vi "士兵升变.vi"(2 "选项":enum16{"士兵", "骑士", "主教", "战车", "皇后"}(ring), 3 "到达的Y":u8, 4 "到达的X":u8, 5 "输入的棋盘":T1) -> (0 "输出棋盘":T1, 1 "数值":u8)   [LabVIEW 2017]
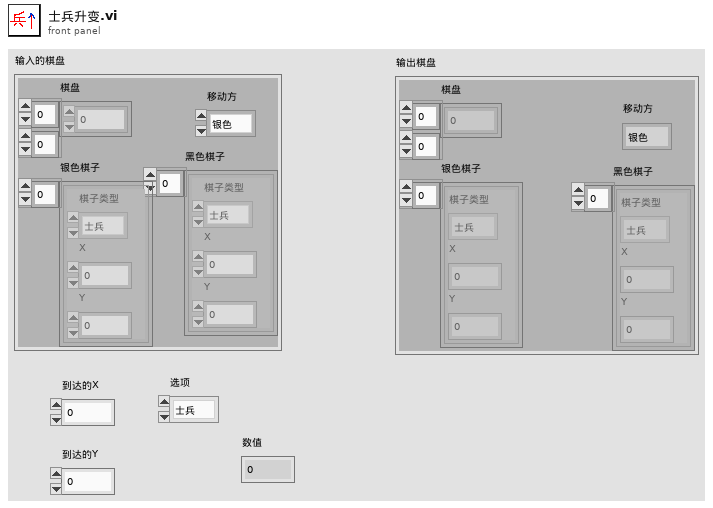
[diagram p1: front panel]
types:
  T1 = cluster{"棋盘":u16[][], "银色棋子":cluster{"棋子类型":enum16{"士兵", "骑士", "主教", "战车", "皇后", "国王", "空"}, "X":u8, "Y":u8}[], "黑色棋子":cluster{"棋子类型":enum16{"士兵", "骑士", "主教", "战车", "皇后", "国王", "空"}, "X":u8, "Y":u8}[], "移动方":enum16{"银色", "黑色"}}
  T2 = cluster{"棋子类型":enum16{"士兵", "骑士", "主教", "战车", "皇后", "国王", "空"}, "X":u8, "Y":u8}[]
  T3 = cluster{"y":enum16{"士兵", "骑士", "主教", "战车", "皇后", "国王", "空"}, "到达的X":u8, "到达的Y":u8}
  T4 = cluster{"棋子类型":enum16{"士兵", "骑士", "主教", "战车", "皇后", "国王", "空"}, "到达的X":u8, "到达的Y":u8}
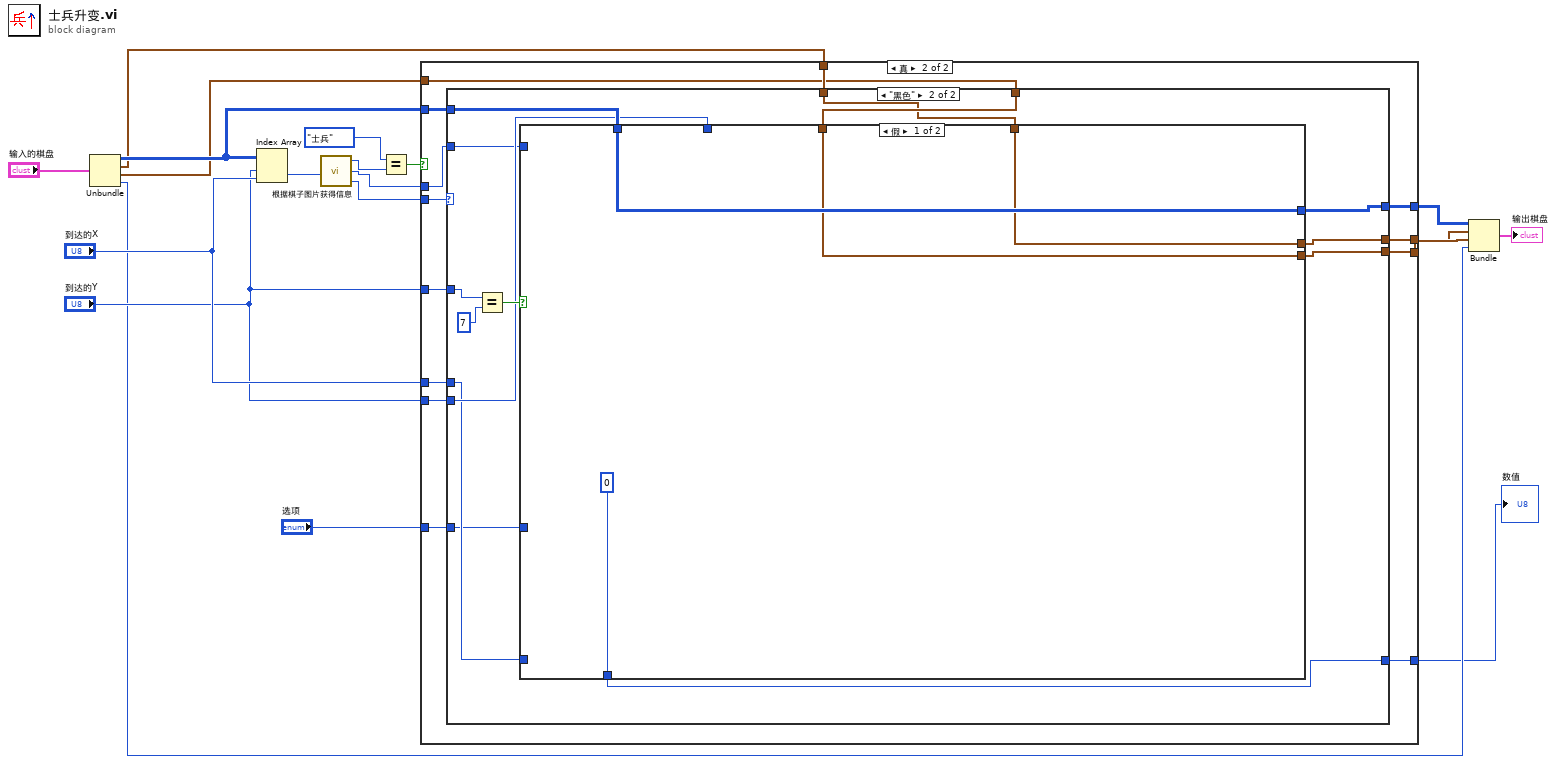
[diagram p0: block diagram]
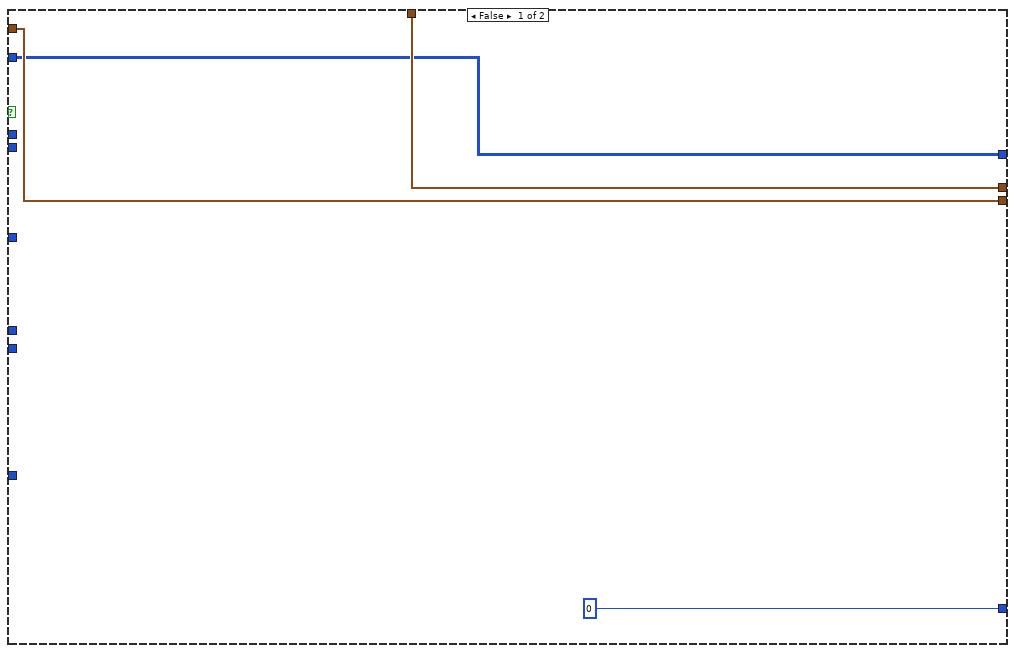
[diagram p2: hidden frame]
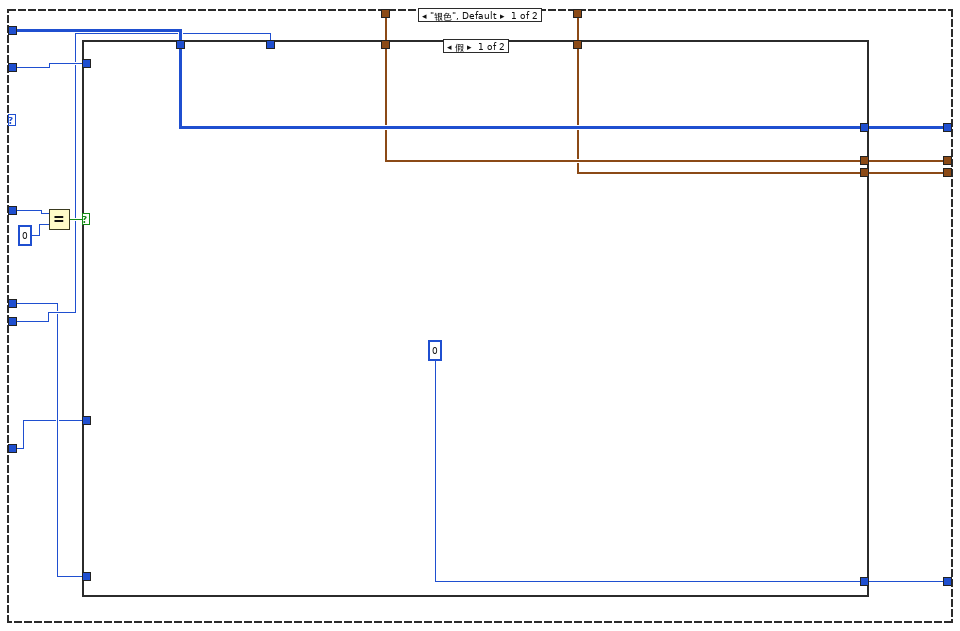
[diagram p3: hidden frame]
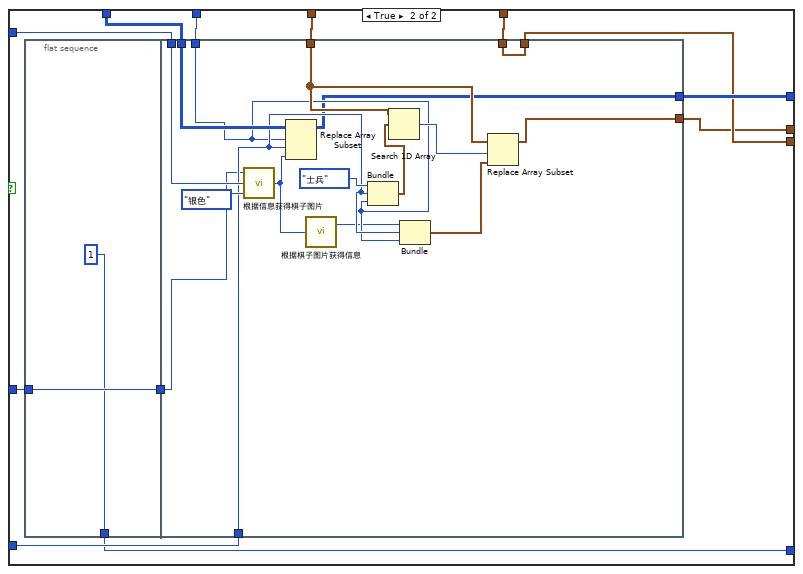
[diagram p4: hidden frame]
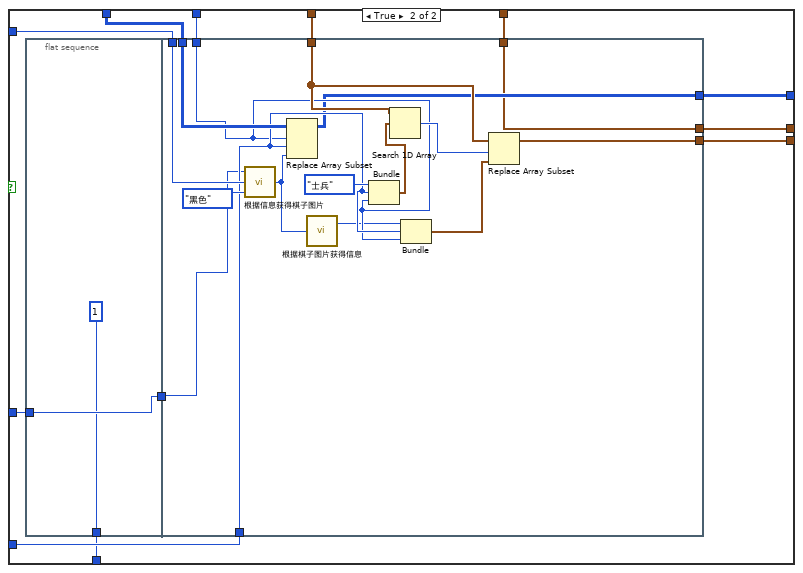
[diagram p5: hidden frame]
diagram:
  n1 = Unbundle("输入的棋盘") -> ("棋盘"=w14:u16[][], "银色棋子"=w9:T2, "黑色棋子"=w8:T2, "移动方"=w6:enum16{"银色", "黑色"})
  n2 = Index Array(array=w14, index (row)="到达的Y", index (col)="到达的X") -> (element=w18:u16)
  n3 = call "根据棋子图片获得信息.vi"("棋子"=w18) -> ("棋子类型"=w17:enum16{"士兵", "骑士", "主教", "战车", "皇后", "国王", "空"}, "背景颜色"=w11:enum16{"白色", "绿色"}, "棋子颜色"=w10:enum16{"银色", "黑色"})
  n4 = Equal?(x=enum16{"士兵", "骑士", "主教", "战车", "皇后", "国王", "空"}."士兵" ("y"), y=w17) -> (x = y?=w15:bool)
  n5 = case shown="真" w15 {
    tunnel: w10 -> [_ w36]
    tunnel: "到达的Y" -> [_ w35]
    tunnel: w14 -> [w21 w34]
    tunnel: "到达的X" -> [_ w33]
    tunnel: "到达的Y" -> [_ w32]
    tunnel: w11 -> [_ w31]
    tunnel: w9 -> [w23 w30]
    tunnel: w8 -> [w22 w29]
    tunnel: [w22 w27] -> w4
    tunnel: [w21 w28] -> w7
    tunnel: [w23 w26] -> w3
    tunnel: "选项" -> [_ w25]
    tunnel: [0 w24] -> w1
    frame False {
    }
    frame True {
      n6 = case shown="\"黑色\"" w36 {
        tunnel: w35 -> [w50 w97]
        tunnel: w34 -> [w47 w95]
        tunnel: w33 -> [w44 w92]
        tunnel: w32 -> [w45 w94]
        tunnel: w31 -> [w46 w93]
        tunnel: w30 -> [w43 w90]
        tunnel: w29 -> [w42 w91]
        tunnel: [w40 w87] -> w27
        tunnel: [w41 w89] -> w28
        tunnel: [w39 w88] -> w26
        tunnel: w25 -> [w38 w86]
        tunnel: [w37 w85] -> w24
        frame "银色", Default {
          n7 = Equal?(x=w50, y=u8 0) -> (x = y?=w48:bool)
          n8 = case shown="假" w48 {
            tunnel: w47 -> [w54 w66]
            tunnel: w46 -> [_ w65]
            tunnel: w45 -> [_ w64]
            tunnel: w44 -> [_ w63]
            tunnel: w43 -> [w53 w62]
            tunnel: w42 -> [w52 w61]
            tunnel: [w52 w59] -> w40
            tunnel: [w54 w60] -> w41
            tunnel: [w53 w58] -> w39
            tunnel: w38 -> [_ w56]
            tunnel: [0 w55] -> w37
            frame False {
            }
            frame True {
              n9 = flat-sequence {
                tunnel: [w68] -> w57
                tunnel: w56 -> [w68]
                tunnel: [1] -> w55
                tunnel: w66 -> [w84]
                tunnel: w65 -> [w83]
                tunnel: w64 -> [w75]
                tunnel: w63 -> [w76]
                tunnel: w62 -> [w79]
                tunnel: w61 -> [w71]
                tunnel: [w71] -> w59
                tunnel: [w72] -> w60
                tunnel: [w70] -> w58
                tunnel: w57 -> [w69]
                frame #0 {
                }
                frame #1 {
                  n10 = call "根据信息获得棋子图片.vi"("棋子颜色"=enum16{"银色", "黑色"}."银色", "背景颜色"=w83, "棋子类型"=w69) -> ("棋子"=w77:u16)
                  n11 = Replace Array Subset(array=w84, new element=w77, index (row)=w75, index (col)=w76) -> (w72:u16[][])
                  n12 = call "根据棋子图片获得信息.vi"("棋子"=w77) -> ("棋子类型"=w74:enum16{"士兵", "骑士", "主教", "战车", "皇后", "国王", "空"})  [unwired: 2 out]
                  n13 = Bundle("y"=enum16{"士兵", "骑士", "主教", "战车", "皇后", "国王", "空"}."士兵", "到达的X"=w76, "到达的Y"=w75) -> (w80:T3)  [unwired: 1 in]
                  n14 = Search 1D Array(1D array=w79, element=w80) -> (index of element=w78:i32)  [unwired: 1 in]
                  n15 = Bundle("棋子类型"=w74, "到达的X"=w76, "到达的Y"=w75) -> (w73:T4)  [unwired: 1 in]
                  n16 = Replace Array Subset(array=w79, new element=w73, index=w78) -> (w70:T2)
                }
              }
            }
          }
        }
        frame "黑色" {
          n17 = Equal?(x=w97, y=u8 7) -> (x = y?=w98:bool)
          n18 = case shown="假" w98 {
            tunnel: w95 -> [w102 w114]
            tunnel: w93 -> [_ w113]
            tunnel: w94 -> [_ w112]
            tunnel: w92 -> [_ w111]
            tunnel: w91 -> [w100 w110]
            tunnel: w90 -> [w101 w109]
            tunnel: [w100 w108] -> w87
            tunnel: [w102 w107] -> w89
            tunnel: [w101 w106] -> w88
            tunnel: w86 -> [_ w105]
            tunnel: [0 w103] -> w85
            frame False {
            }
            frame True {
              n19 = flat-sequence {
                tunnel: w105 -> [w116]
                tunnel: [w116] -> w104
                tunnel: [1] -> w103
                tunnel: w114 -> [w132]
                tunnel: w113 -> [w131]
                tunnel: w112 -> [w123]
                tunnel: w111 -> [w124]
                tunnel: w110 -> [w127]
                tunnel: w109 -> [w118]
                tunnel: [w120] -> w108
                tunnel: [w119] -> w107
                tunnel: [w118] -> w106
                tunnel: w104 -> [w117]
                frame #0 {
                }
                frame #1 {
                  n20 = call "根据信息获得棋子图片.vi"("棋子颜色"=enum16{"银色", "黑色"}."黑色", "背景颜色"=w131, "棋子类型"=w117) -> ("棋子"=w125:u16)
                  n21 = Replace Array Subset(array=w132, new element=w125, index (row)=w123, index (col)=w124) -> (w119:u16[][])
                  n22 = call "根据棋子图片获得信息.vi"("棋子"=w125) -> ("棋子类型"=w122:enum16{"士兵", "骑士", "主教", "战车", "皇后", "国王", "空"})  [unwired: 2 out]
                  n23 = Bundle("y"=enum16{"士兵", "骑士", "主教", "战车", "皇后", "国王", "空"}."士兵", "到达的X"=w124, "到达的Y"=w123) -> (w128:T3)  [unwired: 1 in]
                  n24 = Search 1D Array(1D array=w127, element=w128) -> (index of element=w126:i32)  [unwired: 1 in]
                  n25 = Bundle("棋子类型"=w122, "到达的X"=w124, "到达的Y"=w123) -> (w121:T4)  [unwired: 1 in]
                  n26 = Replace Array Subset(array=w127, new element=w121, index=w126) -> (w120:T2)
                }
              }
            }
          }
        }
      }
    }
  }
  "数值" <- w1
  n27 = Bundle("棋盘"=w7, "银色棋子"=w3, "黑色棋子"=w4, "移动方"=w6) -> (→"输出棋盘":T1)  [unwired: 1 in]
